vi "Reset Wifi.vi"(7 "Retry wait time [ms]":u32=200, 8 "error in (no error)":errorcluster, 10 "Hard Reset?":bool, 11 "LINX Resource":T1) -> (0 "error out":errorcluster, 1 "Connected?":bool, 2 "TCP Config":T5, 3 "LINX Resource Out":T1)   [LabVIEW 2019, in "LINXx.lvlib"]
doc: "Resets WiFi connection; select Hard boolean to reboot entire board and reconnect"
uses:
  LINXx.lvlib
  <vilib>/MakerHub/LINX/Private/Type Defs/LINX Ref.ctl
  <vilib>/MakerHub/LINX/Private/Type Defs/Platform.ctl
  <vilib>/MakerHub/LINX/Private/Type Defs/Interface.ctl
  <vilib>/MakerHub/LINX/Private/Device/Type Defs/LINX Device Config.ctl
  <vilib>/MakerHub/LINX/Private/Device/Type Defs/TCP Config.ctl
  <vilib>/MakerHub/LINX/Private/Device/Type Defs/Channels.ctl
  Public/Reset Target.ctl
  WiFi101 Status.ctl
  <vilib>/MakerHub/LINX/LMH-LINX.lvlib
  <vilib>/MakerHub/LINX/Private/Device/Device.lvlib
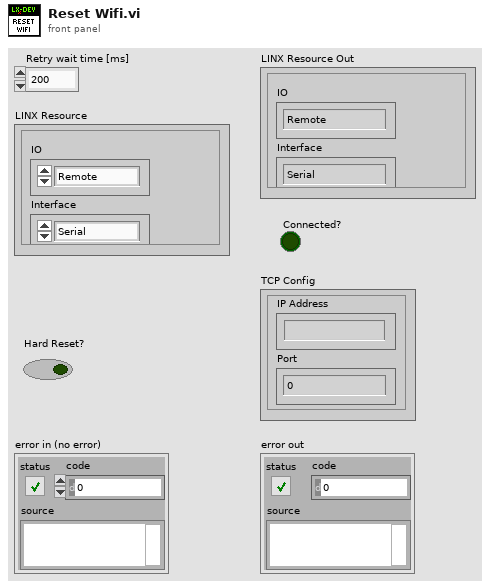
[diagram p1: front panel]
types:
  T1 = typedef "LMH-LINX.lvlib/LINX Ref.ctl" = cluster{"IO":T2, "Interface":T3, "LINX Device Config":T4}
  T2 = typedef "LMH-LINX.lvlib/Platform.ctl" = enum16{"Remote", "Local"}
  T3 = typedef "LMH-LINX.lvlib/Interface.ctl" = enum16{"Serial", "TCP"}
  T4 = typedef "LMH-LINX.lvlib/Device.lvlib/LINX Device Config.ctl" = cluster{"Interface":T3, "COM Port":refnum<visa-resource-name>, "TCP Configuration":T5, "Device Family":u8, "Device ID":u8, "Device Name":string, "TCP Ref":refnum<k5>, "Channels":T6}
  T5 = typedef "LMH-LINX.lvlib/Device.lvlib/TCP Config.ctl" = cluster{"IP Address":string, "Port":u16}
  T6 = typedef "LMH-LINX.lvlib/Channels.ctl" = cluster{"DI":u8[], "DO":u8[], "AI":u8[], "AO":u8[], "PWM":u8[], "QE":u8[], "UART":u8[], "I2C 2":u8[], "SPI":u8[], "CAN":u8[], "Servo":u8[], "AI Ref (V)":dbl, "AI Resolution (Bits)":u8, "AO Ref (V)":dbl, "AO Resolution (Bits)":u8}
  T7 = typedef "LINXx.lvlib/Reset Target.ctl" = enum16{"None", "Serial", "TCP", "Board"}
  T8 = typedef "LINXx.lvlib/WiFi101 Status.ctl" = u8
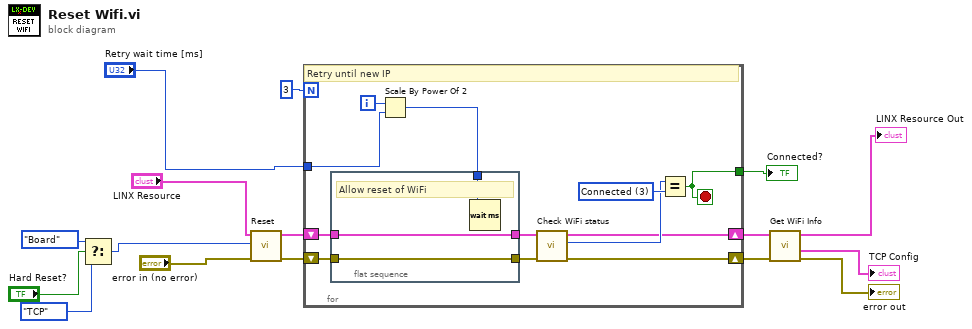
[diagram p0: block diagram]
diagram:
  n1 = Select(t=Reset_Target."Board" ("Reset Target"), s="Hard Reset?", f=Reset_Target."TCP") -> (s? t:f=w3:T7)
  n2 = call "Reset.vi"("Error In"="error in (no error)", "Reset Target"=w3, "LINX Resource"="LINX Resource") -> ("Error Out"=w13:errorcluster, "LINX Resource out"=w12:T1)  [unwired: 7 in]
  n3 = for {
    N: 3 -> [_]
    shift-right: [w20] -> w6
    shift-left: w12 -> [w27]
    shift-right: [w23] -> w8
    shift-left: w13 -> [w26]
    tunnel: [w28] -> w11
    tunnel: "Retry wait time [ms]" -> [w18]
    i -> [w19]
    stop <- w28 stop-if-true
    w22 = T8 3 items=["No module"=255, "Idle"=0, "No SSID"=1, "Scan completed"=2, "Connected"=3, "Connection failed"=4, "Connection lost"=5, "Disconnected"=6, "AP listening"=7, "AP connected"=8, "AP failed"=9, "Provisioning"=10, "Provisioning failed"=11] ("Ring")
    # "Retry until new IP"
    n4 = flat-sequence {
      tunnel: w27 -> [w31]
      tunnel: [w31] -> w25
      tunnel: w26 -> [w30]
      tunnel: [w30] -> w24
      tunnel: w17 -> [w29]
      frame #0 {
        # "Allow reset of WiFi"
        n5 = Wait (ms)(milliseconds to wait=w29) -> ()  [unwired: 1 out]
      }
    }
    n6 = Scale By Power Of 2(n=w19, x=w18) -> (x*2^n=w17:u32)
    n7 = call "Check WiFi status.vi"("Error In"=w24, "LINX Resource"=w25) -> ("Error Out"=w23:errorcluster, "WiFi status"=w21:u8, "LINX Resource out"=w20:T1)  [unwired: 7 in]
    n8 = Equal?(x=w21, y=w22) -> (x = y?=w28:bool)
  }
  "Connected?" <- w11
  n9 = call "Get WiFi Info.vi"("Error In"=w8, "LINX Resource"=w6) -> ("Error Out"=→"error out":errorcluster, "TCP Config"=→"TCP Config":T5, "LINX Resource Out"=→"LINX Resource Out":T1)  [unwired: 6 in, 1 out]
